vi "Config-Sampling-Parameters.vi"(0 "VISA session":refnum<visa-resource-name>, 1 "mode (linear: 0)":i32(ring) items=["linear", "log 10", "log 25", "log 50", "thinned out"], 3 "initial interval (sec)":dbl=0.004 format="%^.3e", 4 "sampling time\n(linear/thinned-out only)":i32(ring) items=["auto (linear only)", "no limit", "set limit "], 5 "number of samples":i32=1, 7 "error in (no error)":errorcluster, 8 "sampling time limit":dbl=10.0 format="%.1f", 9 "filter status":bool, 10 "num. of events":i32=1, 11 "event (val > threshold:0)":i32(ring) items=["Value > Threshold", "Value < Threshold", "| Value | > | Threshold |", "| Value | < | Threshold |"], 12 "stop condition":bool, 13 "hold time (sec)":dbl format="%.4f", 14 "enable delay":dbl format="%.1f", 15 "output sequence mode":bool, 16 "name":string, 17 "threshold":dbl format="%^.2e") -> (20 "VISA resource name out":refnum<visa-resource-name>, 27 "error out":errorcluster)   [LabVIEW 2016, in "Agilent 415X Series.lvlib"]
doc: "This VI confiures sampling measurement parameters.\n\n* This VI does not check whether the instrument is placed in SAMPLING mode. To set the instrument's measurement mode, run HP415xA Select Measurement Mode.vi."
uses:
  Agilent 415X Series.lvlib
panel:
  # "on\noff"
  # "(sec)"
  # "enable\ndisable"
  # "(sec)"
  # "sequential\nsimultaneous"
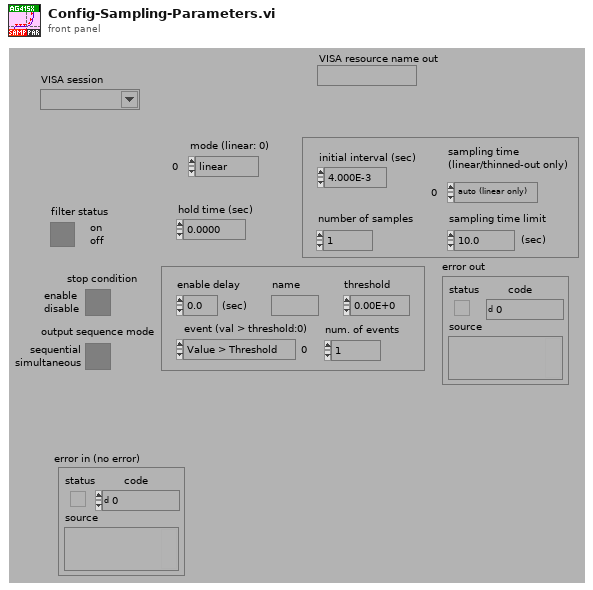
[diagram p1: front panel]
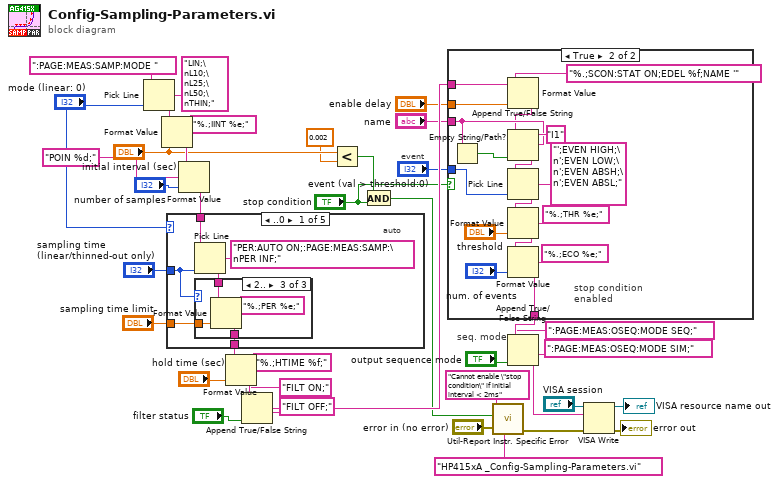
[diagram p0: block diagram]
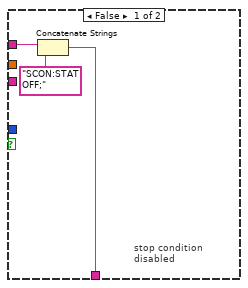
[diagram p2: hidden frame]
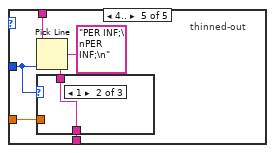
[diagram p8: hidden frame]
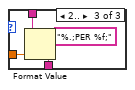
[diagram p10: hidden frame]
diagram:
  # "seq. mode"
  # "event"
  n1 = Pick Line(string ("")=":PAGE:MEAS:SAMP:MODE ", multi-line string="LIN;\nL10;\nL25;\nL50;\nTHIN;", line index="mode (linear: 0)") -> (output string=w34:string)
  n2 = Format Value(string ("")=w34, format string="%.;IINT %e;", value (0)="initial interval (sec)") -> (output string=w35:string)
  n3 = Format Value(string ("")=w35, format string="POIN %d;", value (0)="number of samples") -> (output string=w30:string)
  n4 = case shown="..0" "mode (linear: 0)" {
    tunnel: "sampling time\n(linear/thinned-out only)" -> [w43 _ _ _ w58]
    tunnel: w30 -> [w45 w52 w53 w54 w60]
    tunnel: "sampling time limit" -> [w41 _ _ _ w56]
    tunnel: [w40 w52 w53 w54 w55] -> w27
    frame ..0 {
      # "auto"
      n5 = Pick Line(string ("")=w45, multi-line string="PER:AUTO ON;:PAGE:MEAS:SAMP:\nPER INF;", line index=w43) -> (output string=w42:string)
      n6 = case shown="2.." w43 {
        tunnel: w42 -> [w46 w47 w50]
        tunnel: w41 -> [_ _ w49]
        tunnel: [w46 w47 w48] -> w40
        frame ..0 {
        }
        frame 1 {
        }
        frame 2.. {
          n7 = Format Value(string ("")=w50, format string="%.;PER %e;", value (0)=w49) -> (output string=w48:string)
        }
      }
    }
    frame 1 {
      # "log 10"
    }
    frame 2 {
      # "log 25"
    }
    frame 3 {
      # "log 50"
    }
    frame 4.. {
      # "thinned-out"
      n8 = Pick Line(string ("")=w60, multi-line string="PER INF;\nPER INF;\n", line index=w58) -> (output string=w57:string)
      n9 = case shown="1" w58 {
        tunnel: w57 -> [w61 w62 w65]
        tunnel: w56 -> [_ _ w64]
        tunnel: [w61 w62 w63] -> w55
        frame ..0 {
        }
        frame 1 {
        }
        frame 2.. {
          n10 = Format Value(string ("")=w65, format string="%.;PER %f;", value (0)=w64) -> (output string=w63:string)
        }
      }
    }
  }
  n11 = Format Value(string ("")=w27, format string="%.;HTIME %f;", value (0)="hold time (sec)") -> (output string=w25:string)
  n12 = Append True/False String(1:"filter status", 2:"FILT OFF;", 3:"FILT ON;", 4:w25) -> (0:w18:string)
  n13 = Less?(x="initial interval (sec)", y=0.002) -> (x < y?=w19:bool)
  n14 = And(x=w19, y="stop condition") -> (x .and. y?=w8:bool)
  n15 = case shown="True" "stop condition" {
    tunnel: w18 -> [w69 w85]
    tunnel: "enable delay" -> [_ w84]
    tunnel: "name" -> [_ w80]
    tunnel: "event (val > threshold:0)" -> [_ w78]
    tunnel: [w67 w71] -> w6
    frame False {
      # "stop condition \ndisabled"
      n16 = Concatenate Strings(w69, "SCON:STAT OFF;") -> (w67:string)
    }
    frame True {
      # "stop condition \nenabled"
      n17 = Empty String/Path?(string/path=w80) -> (empty?=w81:bool)
      n18 = Format Value(string ("")=w85, format string="%.;SCON:STAT ON;EDEL %f;NAME '", value (0)=w84) -> (output string=w77:string)
      n19 = Append True/False String(1:w81, 2:w80, 3:"I1", 4:w77) -> (0:w79:string)
      n20 = Pick Line(string ("")=w79, multi-line string="';EVEN HIGH;\n';EVEN LOW;\n';EVEN ABSH;\n';EVEN ABSL;", line index=w78) -> (output string=w76:string)
      n21 = Format Value(string ("")=w76, format string="%.;THR %e;", value (0)="threshold") -> (output string=w73:string)
      n22 = Format Value(string ("")=w73, format string="%.;ECO %e;", value (0)="num. of events") -> (output string=w71:string)
    }
  }
  n23 = call "Util-Report Instr. Specific Error.vi"("source"="HP415xA _Config-Sampling-Parameters.vi", "error in (no error)"="error in (no error)", "error message"="Cannot enable \"stop condition\" if initial interval < 2ms", "new error"=w8) -> ("error out"=w9:errorcluster)  [unwired: 6 in, 1 out]
  n24 = Append True/False String(1:"output sequence mode", 2:":PAGE:MEAS:OSEQ:MODE SIM;", 3:":PAGE:MEAS:OSEQ:MODE SEQ;", 4:w6) -> (0:w5:string)
  n25 = VISA Write(VISA resource name="VISA session", write buffer=w5, error in (no error)=w9) -> (VISA resource name out=→"VISA resource name out":refnum<visa-resource-name>, error out=→"error out":errorcluster)  [unwired: 1 out]
